vi "DS读属性数据.vi"() -> ()   [LabVIEW 2010]
panel:
  in  "停止":bool
  out "变体数据":variant
  out "数据发送时间":string
  out "波形图":dbl[](graph)
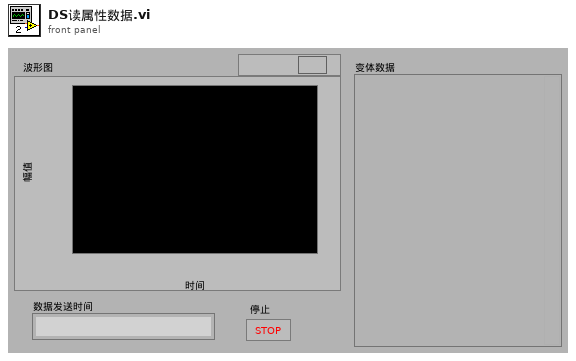
[diagram p1: front panel]
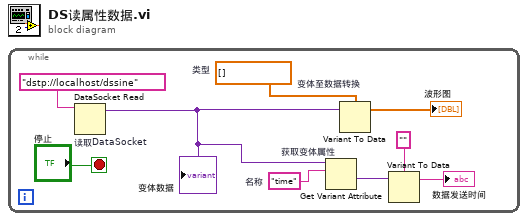
[diagram p0: block diagram]
diagram:
  n1 = while {
    stop <- "停止" stop-if-true
    w3 = "time"  # 名称
    w8 = dbl[] []  # 类型
    n2 = DataSocket Read "读取DataSocket"(11:"dstp://localhost/dssine" ("URL")) -> (2:w4:variant)  [unwired: 4 in, 6 out]
    "变体数据" <- w4
    n3 = Get Variant Attribute "获取变体属性"(Variant=w4, name=w3) -> (value=w2:variant)  [unwired: 2 in, 3 out]
    n4 = Variant To Data "变体至数据转换"(Variant=w4, type=w8) -> (data=→"波形图":dbl[])  [unwired: 1 in, 1 out]
    n5 = Variant To Data(Variant=w2, type="") -> (data=→"数据发送时间":string)  [unwired: 1 in, 1 out]
  }
